vi "run.vi"(0 "p12":dbl, 5 "p21":dbl, 7 "SNR":dbl) -> (4 "p12":dbl, 8 "p":dbl)   [LabVIEW 2017]
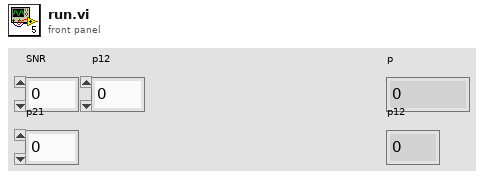
[diagram p1: front panel]
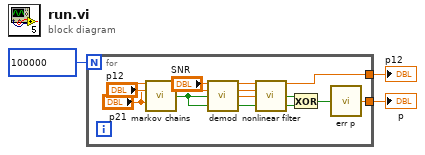
[diagram p0: block diagram]
diagram:
  n1 = for {
    N: 100000 -> [_]
    tunnel: [w5] -> w2
    tunnel: [w4] -> w1
    n2 = call "markov chains.vi"("p12"="p12", "p21"="p21") -> ("bit"=w7:bool)  [unwired: 13 in]
    n3 = call "demod.vi"("SNR"="SNR", "bit"=w7) -> ("soft bit"=w12:dbl)  [unwired: 13 in]
    n4 = call "nonlinear filter.vi"("p12"="p12", "p21"="p21", "soft"=w12) -> ("p12"=w4:dbl, "bit"=w8:bool)  [unwired: 11 in]
    n5 = Exclusive Or(1:w7, 2:w8) -> (0:w6:bool)
    n6 = call "err p.vi"("err"=w6) -> ("p"=w5:dbl)  [unwired: 14 in]
  }
  "p" <- w2
  "p12" <- w1
